vi "ROI grp-Select table cell or entire column.vi"(8 "error in (no error)":errorcluster, 9 "Cell Position":T1, 10 "Button (1=left 2=right)":u16) -> (0 "error out":errorcluster)   [LabVIEW 2020]
uses:
  <vilib>/Utility/miscctls.llb/LVRowAndColumnTypeDef.ctl
  Globals/gl_ROI grp window globals.vi
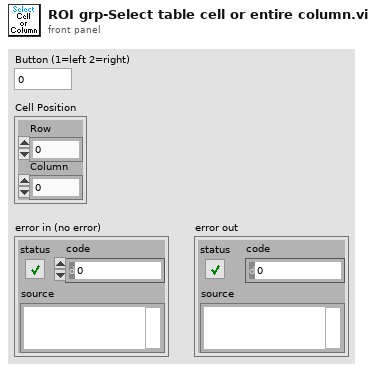
[diagram p1: front panel]
types:
  T1 = typedef "LVRowAndColumnTypeDef.ctl" = cluster{"Row":i32, "Column":i32}
  T2 = typedef "ROI grp-window ctrl refs.ctl" = cluster{"This VI":refnum<vi>, "Pane":refnum<vi>, "Table":refnum<vi>}
  T3 = cluster{"Valid row selected?":bool, "Valid column selected?":bool}
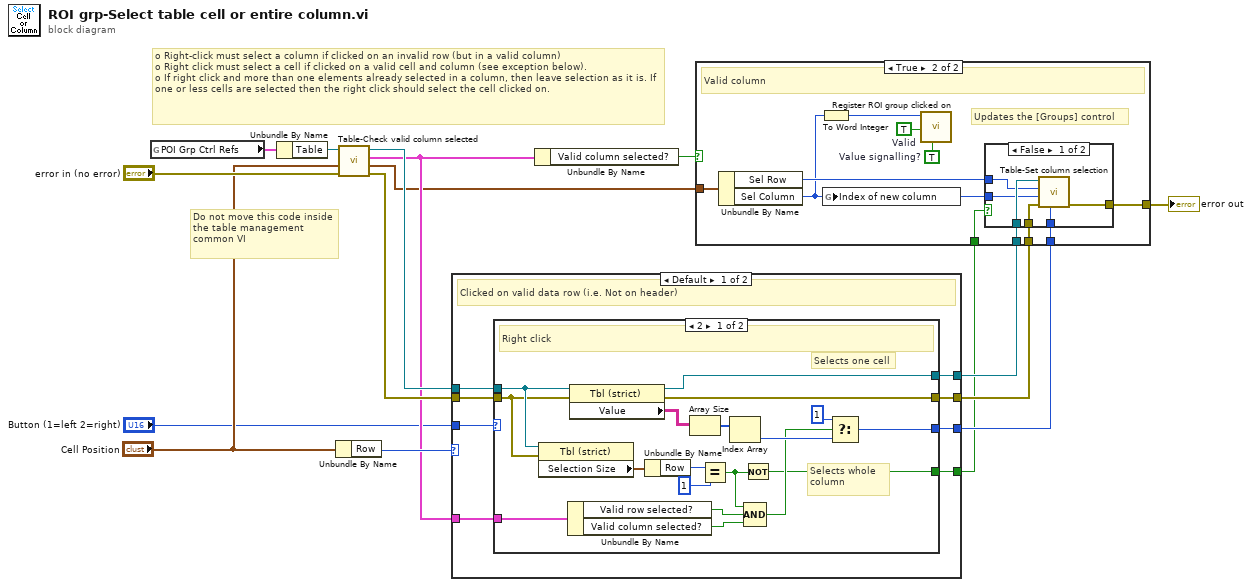
[diagram p0: block diagram]
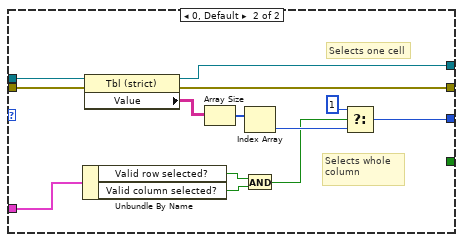
[diagram p2: hidden frame]
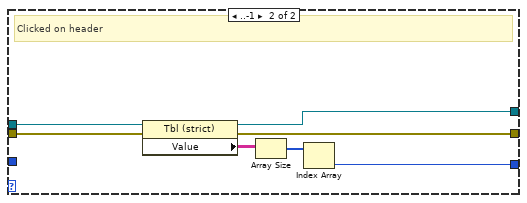
[diagram p3: hidden frame]
diagram:
  # "o\tRight-click must select a column if clicked on an invalid row (but in a valid column)\no\tRight click must select a cell if clicked on a valid cell and column (see exception below).\no\tIf right click and more than one elements already selected in a column, then leave selection as it is. If one or less cells are selected then the right click should select the cell clicked on."
  # "Do not move this code inside the table management common VI"
  n1 = global read "gl_ROI grp window globals.vi" "POI Grp Ctrl Refs"() -> (w1:T2)
  n2 = Unbundle By Name(w1) -> ("Table"=w10:refnum<vi>)
  n3 = Unbundle By Name("Cell Position") -> ("Row"=w9:i32)
  n4 = call <userlib>:"Table-Check valid column selected.vi"("error in (no error)"="error in (no error)", "Cell Position"="Cell Position", "Table ref in"=w10) -> ("error out"=w11:errorcluster, "Selected cell"=w5:cluster{"Sel Row":i32, "Sel Column":i32}, "Selected cell validity cluster"=w6:T3, "Table ref"=w8:refnum<vi>)  [unwired: 4 in, 1 out]
  n5 = case shown="Default" w9 {
    tunnel: [w20 w59] -> w12
    tunnel: w8 -> [w24 w62]
    tunnel: w11 -> [w23 w58]
    tunnel: [w22 w57] -> w14
    tunnel: [w21 w56] -> w13
    tunnel: w6 -> [w19 _]
    tunnel: "Button (1=left 2=right)" -> [w18 _]
    tunnel: [w17 _] -> w2
    frame Default {
      # "Clicked on valid data row (i.e. Not on header)"
      n6 = case shown="2" w18 {
        tunnel: w24 -> [w31 w53]
        tunnel: w23 -> [w30 w52]
        tunnel: [w40 w51] -> w22
        tunnel: [w39 w50] -> w21
        tunnel: [w37 w48] -> w20
        tunnel: w19 -> [w35 w46]
        tunnel: [w25 _] -> w17
        frame 2 {
          # "Selects whole column"
          # "Selects one cell"
          # "Right click"
          n7 = property on="Property Node" class="Tbl (strict)"(reference=w31, error in=w30) -> ("Selection Size"=w29:T1)  [unwired: 2 out]
          n8 = Unbundle By Name(w35) -> ("Valid row selected?"=w34:bool, "Valid column selected?"=w33:bool)
          n9 = property class="Tbl (strict)"(reference=w31, error in=w30) -> (reference out=w39:refnum<vi>, error out=w40:errorcluster, "Value"=w42:string[][])
          n10 = Unbundle By Name(w29) -> ("Row"=w28:i32)
          n11 = Array Size(array=w42) -> (size(s)=w41:i32[])
          n12 = Equal?(x=w28, y=1) -> (x = y?=w26:bool)
          n13 = Index Array(array=w41) -> (element=w36:i32)  [unwired: 1 in]
          n14 = Not(x=w26) -> (.not. x?=w25:bool)
          n15 = Compound Arithmetic op=AND(w26, w34, w33) -> (w32:bool)
          n16 = Select(t=1, s=w32, f=w36) -> (s? t:f=w37:i32)
        }
        frame 0, Default {
          # "Selects whole column"
          # "Selects one cell"
          n17 = Unbundle By Name(w46) -> ("Valid row selected?"=w45:bool, "Valid column selected?"=w44:bool)
          n18 = property class="Tbl (strict)"(reference=w53, error in=w52) -> (reference out=w50:refnum<vi>, error out=w51:errorcluster, "Value"=w55:string[][])
          n19 = Array Size(array=w55) -> (size(s)=w54:i32[])
          n20 = Index Array(array=w54) -> (element=w47:i32)  [unwired: 1 in]
          n21 = And(x=w45, y=w44) -> (x .and. y?=w43:bool)
          n22 = Select(t=1, s=w43, f=w47) -> (s? t:f=w48:i32)
        }
      }
    }
    frame ..-1 {
      # "Clicked on header"
      n23 = property class="Tbl (strict)"(reference=w62, error in=w58) -> (reference out=w56:refnum<vi>, error out=w57:errorcluster, "Value"=w61:string[][])
      n24 = Array Size(array=w61) -> (size(s)=w60:i32[])
      n25 = Index Array(array=w60) -> (element=w59:i32)  [unwired: 1 in]
    }
  }
  n26 = Unbundle By Name(w6) -> ("Valid column selected?"=w7:bool)
  n27 = case shown="True" w7 {
    tunnel: w14 -> [w63 w74]
    tunnel: [w63 w73] -> w16
    tunnel: w13 -> [_ w72]
    tunnel: w12 -> [_ w71]
    tunnel: w5 -> [_ w70]
    tunnel: w2 -> [_ w68]
    frame False {
      # "Invalid column"
    }
    frame True {
      w64 = TRUE  # Value signalling?
      w65 = TRUE  # Valid
      # "Updates the [Groups] control"
      # "Valid column"
      n28 = Unbundle By Name(w70) -> ("Sel Row"=w69:i32, "Sel Column"=w67:i32)
      n29 = To Word Integer(number=w67) -> (16bit integer=w66:i16)
      n30 = global write "gl_ROI grp window globals.vi" "Index of new column"(w67) -> ()
      n31 = call "Register ROI group clicked on.vi"("Value signalling? (F)"=w64, "Valid"=w65, "Group index"=w66) -> ()  [unwired: 7 in, 2 out]
      n32 = case shown="False" w68 {
        tunnel: w74 -> [w80 w81]
        tunnel: [w79 w81] -> w73
        tunnel: w72 -> [w78 _]
        tunnel: w71 -> [w77 _]
        tunnel: w67 -> [w76 _]
        tunnel: w69 -> [w75 _]
        frame False {
          n33 = call <userlib>:"Table-Set column selection.vi"("Selection length (i.e. Number of rows)"=w77, "error in (no error)"=w80, "Index of column to select"=w76, "Index of row to select"=w75, "Table in"=w78) -> ("error out"=w79:errorcluster)  [unwired: 5 in, 1 out]
        }
        frame True {
        }
      }
    }
  }
  "error out" <- w16
